vi "ConnRecoveryThread.vi"(0 "reference in":refnum<class "SuperNS.lvclass">) -> ()   [LabVIEW 2020, in "SuperNS.lvclass"]
doc: "Copyright © 2008 - 2024 VI Technologies B.V. \nALL RIGHTS RESERVED"
uses:
  SuperNS.lvclass
  StreamDataType.ctl
  <vilib>/dex/Flush And Wait Empty Condition.ctl
  <vilib>/Utility/error.llb/Error Cluster From Error Code.vi
  <vilib>/ErrorRing/Error Ring.xnode
  SuperNS.lvclass/SuperNS.ctl
  <resource>/objmgr/ni.dex.rc
panel:
  out "Disconnected timeout":bool
  out "Is Connected":bool
  out "Remote Endpoint Destroyed":bool
  out "Last error":errorcluster
  out "IsWriterEndpoint":bool
  out "Iteration":i32
  # "Copyright (c) 2024, VI Technologies B.V.\nAll rights reserved.\n\nRedistribution and use in source and binary forms, with or without modification, are permitted provided that \nthe following conditions are met:\n\n * Redistributions of source code must retain the above copyright notice, this list of conditions and the \nfollowing disclaimer.\n * Redistributions in binary form must reproduce the above copyright notice, this list of conditions and the \nfollowing disclaimer in the documentation and/or other materials provided with the distribution.\n * Neither the name of VI Technologies B.V. nor the names of its contributors may be used to endorse or \npromote products derived from this software without specific prior written permission.\n\nTHIS SOFTWARE IS PROVIDED BY THE COPYRIGHT HOLDERS AND CONTRIBUTORS \"AS IS\" AND ANY EXPRESS OR \nIMPLIED WARRANTIES, INCLUDING, BUT NOT LIMITED TO, THE IMPLIED WARRANTIES OF MERCHANTABILITY \nAND FITNESS FOR A PARTICULAR PURPOSE ARE DISCLAIMED. IN NO EVENT SHALL THE COPYRIGHT OWNER OR \nCONTRIBUTORS BE LIABLE FOR ANY DIRECT, INDIRECT, INCIDENTAL, SPECIAL, EXEMPLARY, OR CONSEQUENTIAL \nDAMAGES (INCLUDING, BUT NOT LIMITED TO, PROCUREMENT OF SUBSTITUTE GOODS OR SERVICES; LOSS OF \nUSE, DATA, OR PROFITS; OR BUSINESS INTERRUPTION) HOWEVER CAUSED AND ON ANY THEORY OF LIABILITY, \nWHETHER IN CONTRACT, STRICT LIABILITY, OR TORT (INCLUDING NEGLIGENCE OR OTHERWISE) ARISING IN ANY \nWAY OUT OF THE USE OF THIS SOFTWARE, EVEN IF ADVISED OF THE POSSIBILITY OF SUCH DAMAGE.\n\nFor more information, please visit https://www.vi-tech.nl or contact us at info@vi-tech.nl"
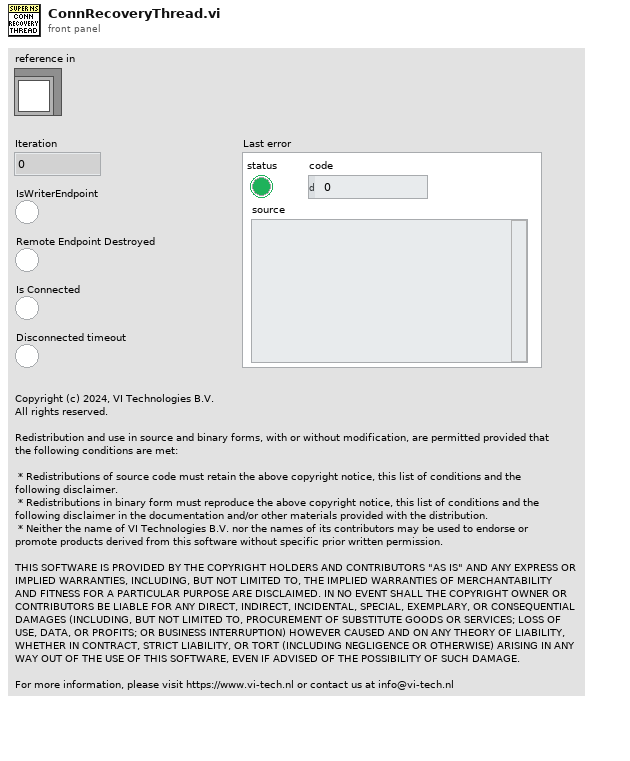
[diagram p1: front panel]
types:
  T1 = typedef "SuperNS.lvclass/ObjectAttributes.ctl" = cluster{"NSName":string, "RemoteEP_URL":string, "BufferSize":i32, "Element Allocation Mode":T2, "ConnLost Timeout":i32, "Writer":bool, "ReadDataEvent":string, "FlushAfterWrite":bool, "Thread":cluster{"VI Refnum":refnum<vi>, "Started Notifier":refnum<notifier>, "Stopped Notifier":refnum<notifier>, "CmdEvent":refnum<user-event>}, "Endpoint":refnum<k21>, "R/W Error":bool, "Flush Wait Condition":T3, "DataReadEvent":refnum<user-event>, "NS Created":bool, "BG ConnCheck/Read period":i32, "ErrorEvent":refnum<user-event>}
  T2 = typedef "Stream Element Allocation Mode.ctl" = u32
  T3 = typedef "Flush And Wait Empty Condition.ctl" = u8
  T4 = typedef "SuperNS.lvclass/StreamDataType.ctl" = refnum<class>
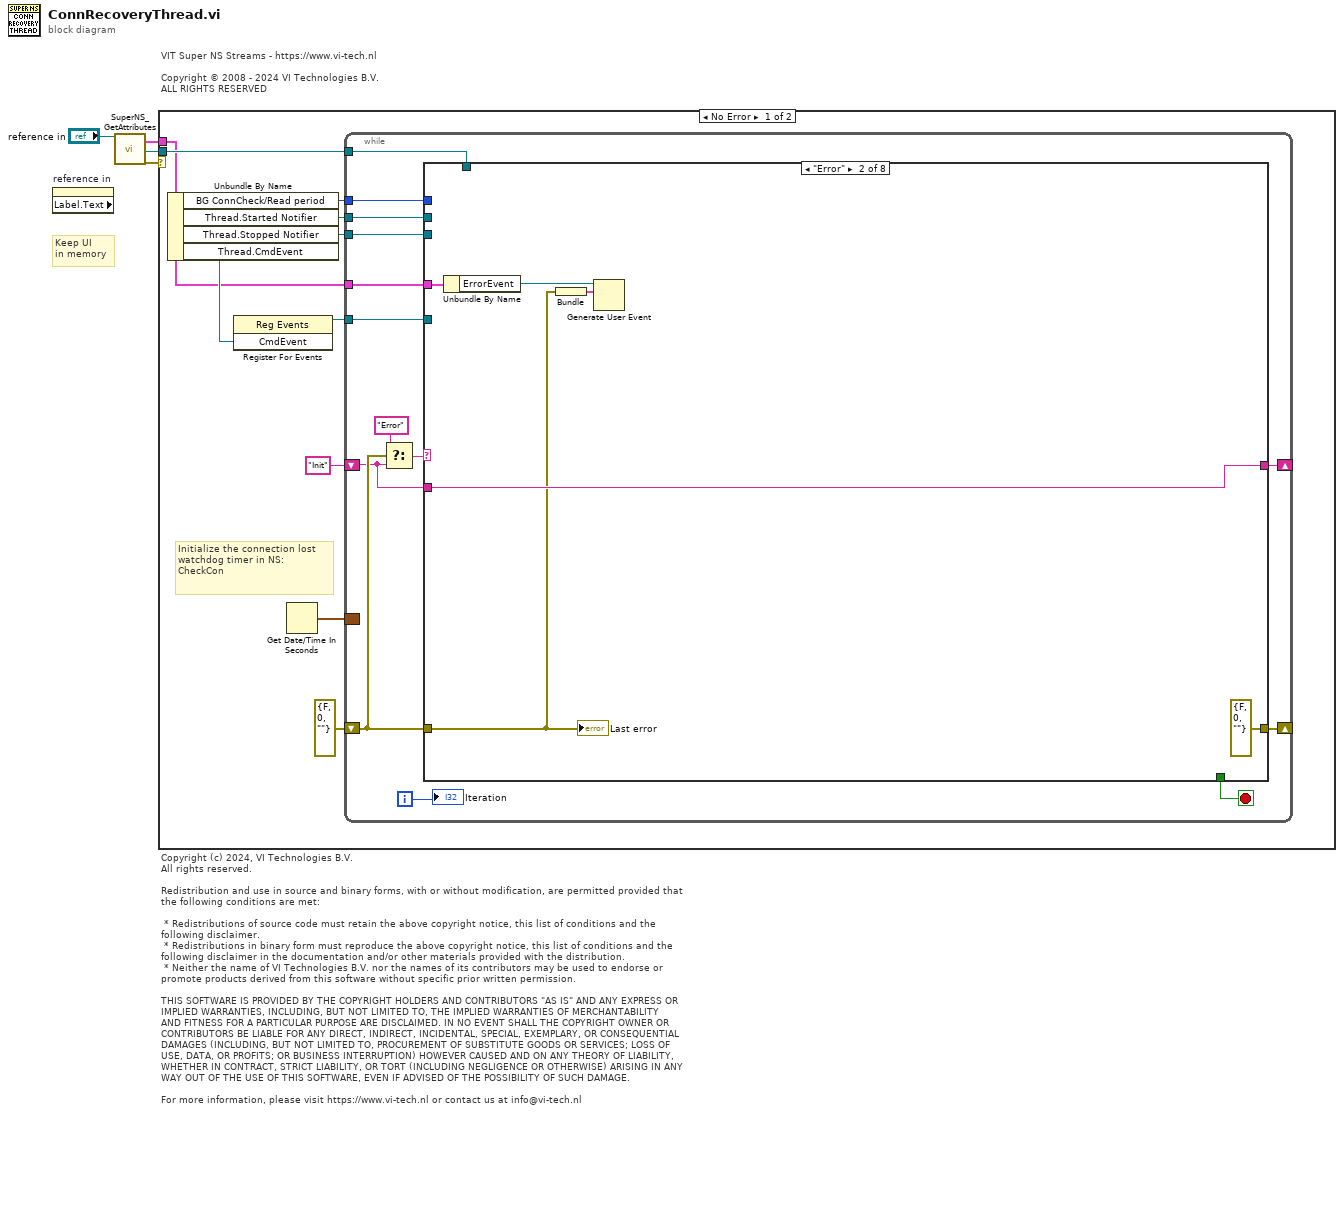
[diagram p0: block diagram]
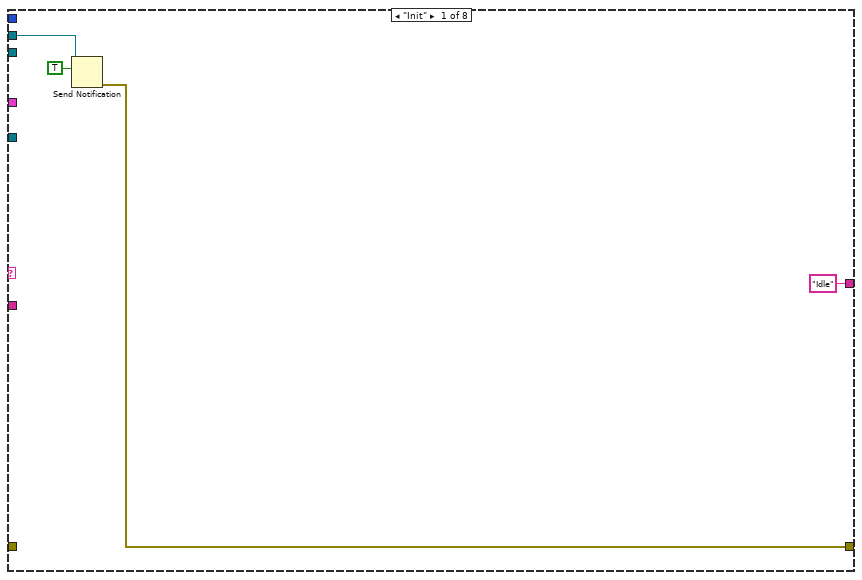
[diagram p2: hidden frame]
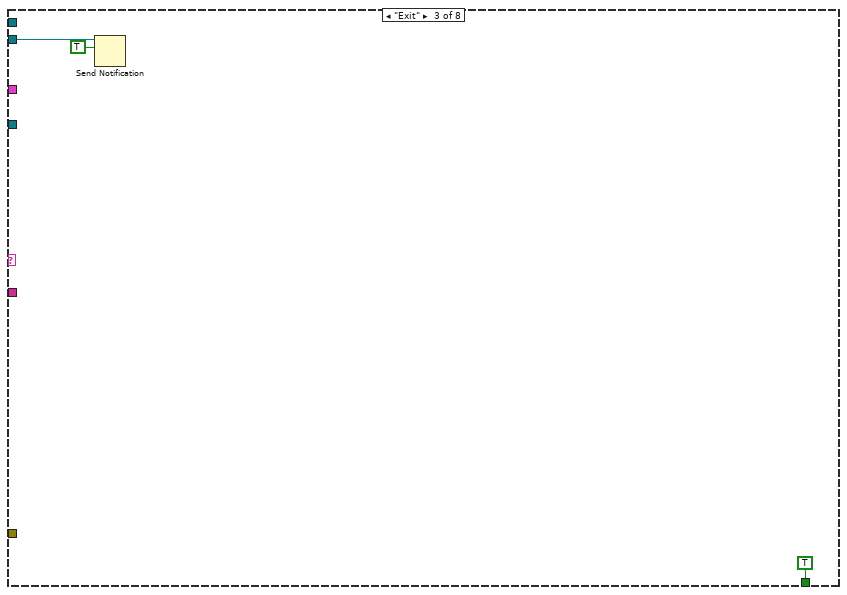
[diagram p3: hidden frame]
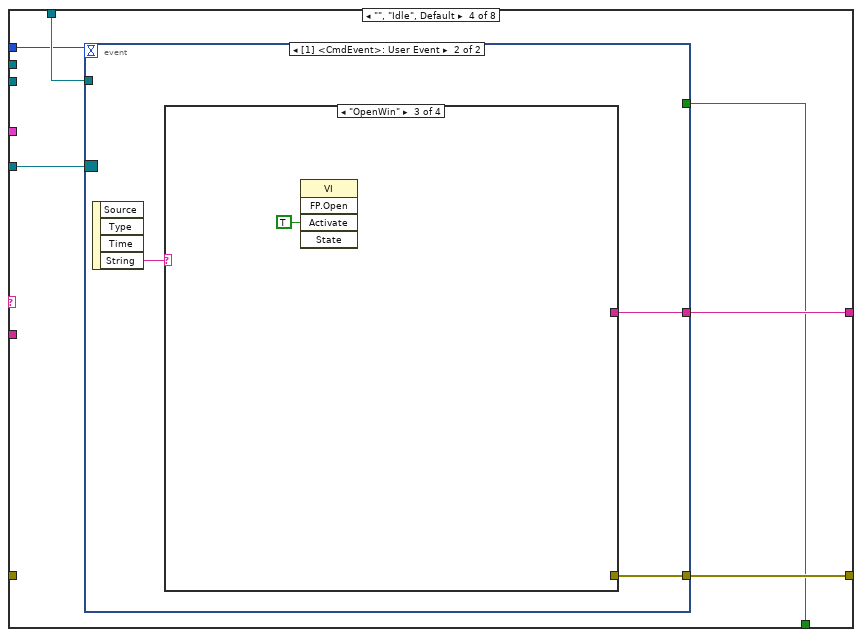
[diagram p4: hidden frame]
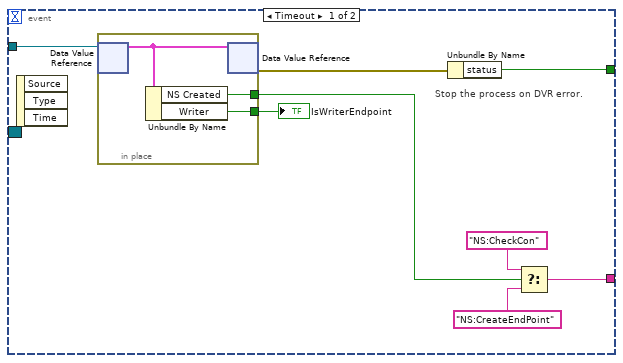
[diagram p5: hidden frame]
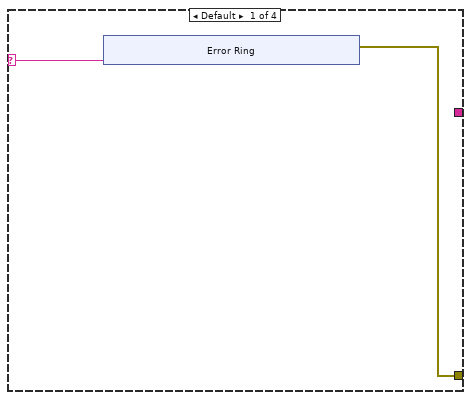
[diagram p6: hidden frame]
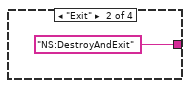
[diagram p7: hidden frame]
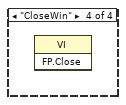
[diagram p8: hidden frame]
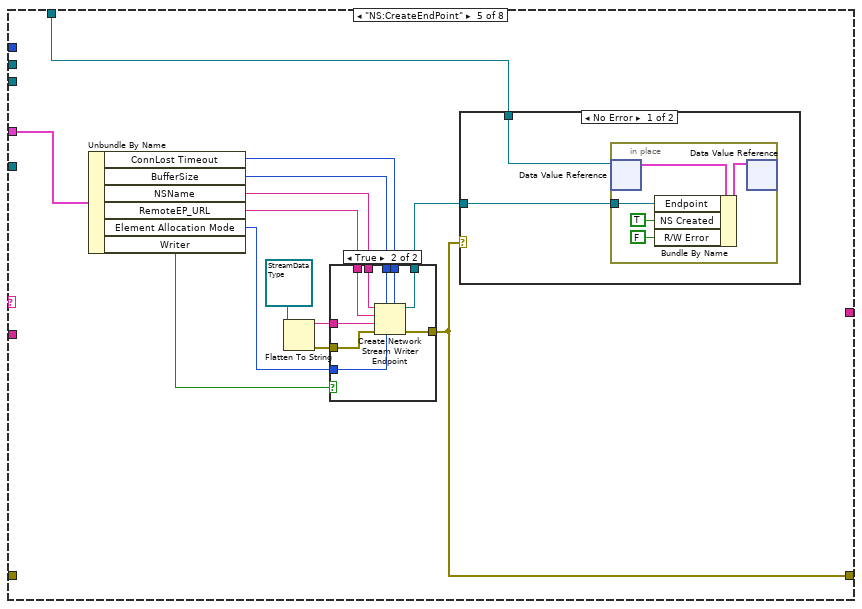
[diagram p9: hidden frame]
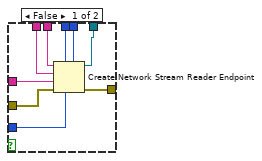
[diagram p10: hidden frame]
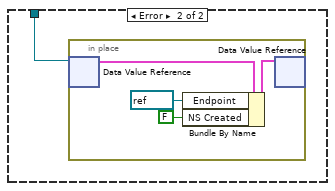
[diagram p11: hidden frame]
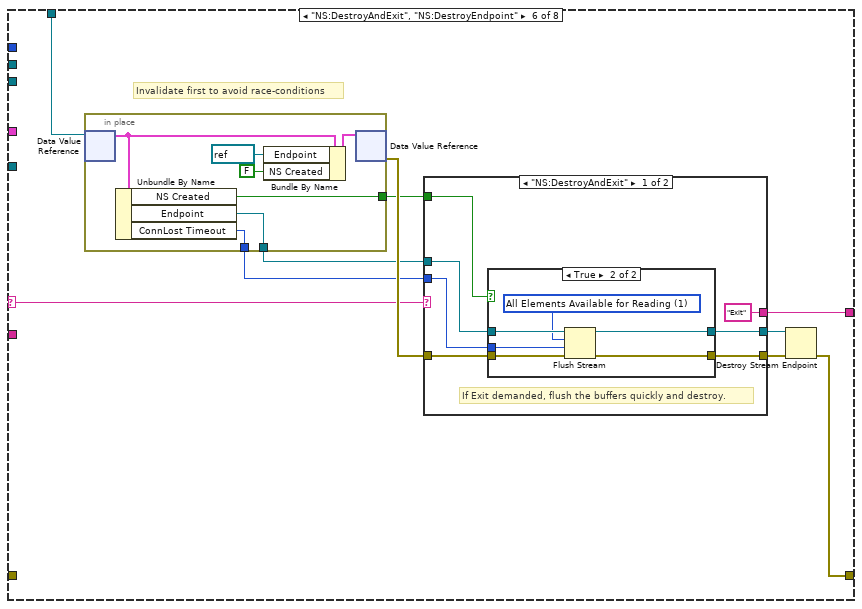
[diagram p12: hidden frame]
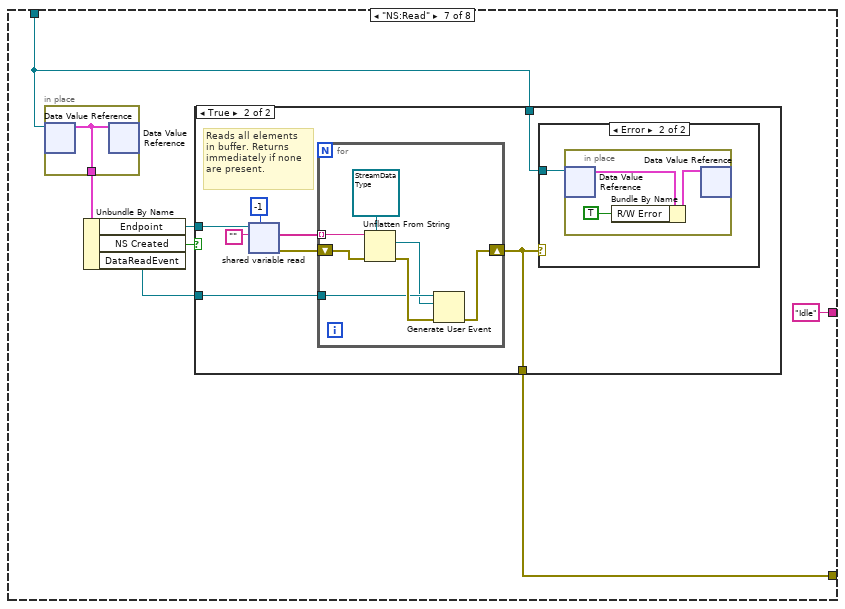
[diagram p15: hidden frame]
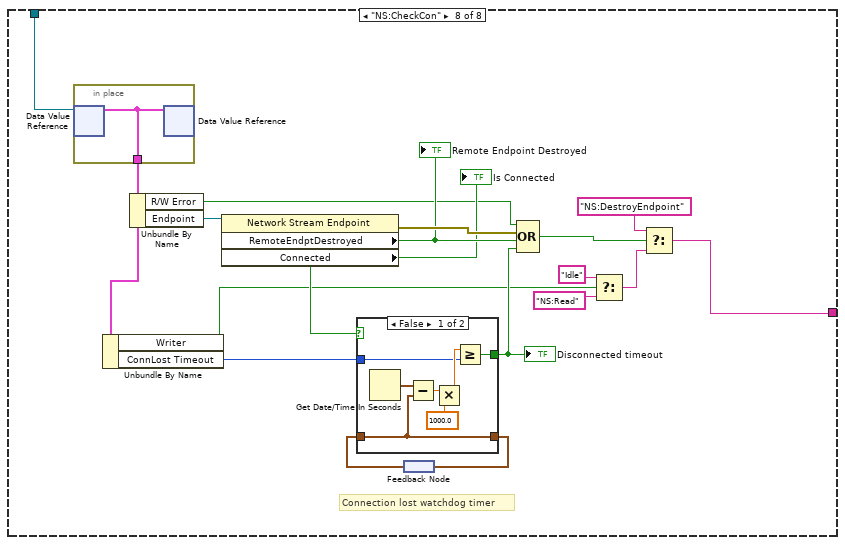
[diagram p18: hidden frame]
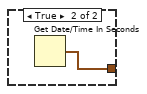
[diagram p19: hidden frame]
diagram:
  # "VIT Super NS Streams - https://www.vi-tech.nl\n\nCopyright © 2008 - 2024 VI Technologies B.V. \nALL RIGHTS RESERVED"
  # "Copyright (c) 2024, VI Technologies B.V.\nAll rights reserved.\n\nRedistribution and use in source and binary forms, with or without modification, are permitted provided that \nthe following conditions are met:\n\n * Redistributions of source code must retain the above copyright notice, this list of conditions and the \nfollowing disclaimer.\n * Redistributions in binary form must reproduce the above copyright notice, this list of conditions and the \nfollowing disclaimer in the documentation and/or other materials provided with the distribution.\n * Neither the name of VI Technologies B.V. nor the names of its contributors may be used to endorse or \npromote products derived from this software without specific prior written permission.\n\nTHIS SOFTWARE IS PROVIDED BY THE COPYRIGHT HOLDERS AND CONTRIBUTORS \"AS IS\" AND ANY EXPRESS OR \nIMPLIED WARRANTIES, INCLUDING, BUT NOT LIMITED TO, THE IMPLIED WARRANTIES OF MERCHANTABILITY \nAND FITNESS FOR A PARTICULAR PURPOSE ARE DISCLAIMED. IN NO EVENT SHALL THE COPYRIGHT OWNER OR \nCONTRIBUTORS BE LIABLE FOR ANY DIRECT, INDIRECT, INCIDENTAL, SPECIAL, EXEMPLARY, OR CONSEQUENTIAL \nDAMAGES (INCLUDING, BUT NOT LIMITED TO, PROCUREMENT OF SUBSTITUTE GOODS OR SERVICES; LOSS OF \nUSE, DATA, OR PROFITS; OR BUSINESS INTERRUPTION) HOWEVER CAUSED AND ON ANY THEORY OF LIABILITY, \nWHETHER IN CONTRACT, STRICT LIABILITY, OR TORT (INCLUDING NEGLIGENCE OR OTHERWISE) ARISING IN ANY \nWAY OUT OF THE USE OF THIS SOFTWARE, EVEN IF ADVISED OF THE POSSIBILITY OF SUCH DAMAGE.\n\nFor more information, please visit https://www.vi-tech.nl or contact us at info@vi-tech.nl"
  # "Keep UI\nin memory"
  n1 = property on="reference in" class="LVClassControl (strict)" props=["Label", "Text"]() -> ()  [unwired: 2 in, 3 out]
  n2 = call "SuperNS_GetAttributes.vi"("reference in"="reference in") -> ("Data"=w1:T1, "DataRef"=w2:refnum<data-value>, "error out"=w4:errorcluster)  [unwired: 15 in, 1 out]
  n3 = case shown="No Error" w4 {
    tunnel: w1 -> [w5 _]
    tunnel: w2 -> [w8 _]
    frame No Error {
      # "Initialize the connection lost watchdog timer in NS: CheckCon"
      n4 = Unbundle By Name(w5) -> ("BG ConnCheck/Read period"=w7:i32, "Thread.Started Notifier"=w9:refnum<notifier>, "Thread.Stopped Notifier"=w11:refnum<notifier>, "Thread.CmdEvent"=w13:refnum<user-event>)
      n5 = register-events(w13) -> (reference out=w12:refnum<event-registration>)  [unwired: 2 in, 1 out]
      n6 = Get Date/Time In Seconds() -> (seconds since 1Jan1904=w6:timestamp)
      n7 = while {
        tunnel: w12 -> [w26]
        tunnel: w11 -> [w25]
        shift-right: [w19] -> _
        shift-left: "Init" -> [w18]
        tunnel: w9 -> [w22]
        shift-right: [w28] -> _
        shift-left: errorcluster {"status"=FALSE, "code"=0, "source"=""} ("error IO") -> [w27]
        tunnel: w8 -> [w17]
        tunnel: w5 -> [w16]
        tunnel: w7 -> [w15]
        border: w6 -> [_]
        i -> [w23]
        stop <- w24 stop-if-true
        n8 = Select(t="Error", s=w27, f=w18) -> (s? t:f=w21:string)
        n9 = case shown="\"Error\"" w21 {
          selector: w21 -> [_ _ _ _ _ w121 _ _]
          tunnel: w26 -> [_ _ _ w46 _ _ _ _]
          tunnel: w25 -> [_ _ w39 _ _ _ _ _]
          tunnel: [_ _ TRUE w42 _ _ _ _] -> w24
          tunnel: w22 -> [w30 _ _ _ _ _ _ _]
          tunnel: [w32 errorcluster {"status"=FALSE, "code"=0, "source"=""} ("error out") _ w47 w84 w123 w156 _] -> w28
          tunnel: ["Idle" w37 _ w45 _ w120 "Idle" w179] -> w19
          tunnel: w18 -> [_ w37 _ _ _ _ _ _]
          tunnel: w17 -> [_ _ _ w44 w73 w119 w151 w178]
          tunnel: w16 -> [_ w36 _ _ w75 _ _ _]
          tunnel: w27 -> [_ w33 _ _ _ _ _ _]
          tunnel: w15 -> [_ _ _ w43 _ _ _ _]
          frame "Init" {
            n10 = Send Notification(notification=TRUE, notifier=w30) -> (error out=w32:errorcluster)  [unwired: 1 in, 1 out]
          }
          frame "Error" {
            n11 = Unbundle By Name(w36) -> ("ErrorEvent"=w35:refnum<user-event>)
            n12 = Bundle("error IO"=w33) -> (w34:cluster{"error IO":errorcluster})  [unwired: 1 in]
            n13 = Generate User Event(user event=w35, event data cluster=w34) -> ()  [unwired: 2 in, 2 out]
            "Last error" <- w33
          }
          frame "Exit" {
            n14 = Send Notification(notification=TRUE, notifier=w39) -> ()  [unwired: 1 in, 2 out]
          }
          frame "", "Idle", Default {
            n15 = event shown="[1] <CmdEvent>: User Event" {
              selector: w46 -> [_ _]
              dyn-events: _ -> [_ _]
              timeout: w43 -> [_ _]
              tunnel: [_ w61] -> w47
              tunnel: [w52 w59] -> w45
              tunnel: w44 -> [w51 _]
              tunnel: [w48 _] -> w42
              event Timeout {
                # "Stop the process on DVR error."
                n16 = event-data() -> ()  [unwired: 1 in, 3 out]
                n17 = in-place {
                  in-place-border: [w57] -> w50
                  in-place-border: [w56] -> w49
                  n18 = in-place-dvr #1(w51) -> (w58:T1)  [unwired: 1 out]
                  n19 = Unbundle By Name(w58) -> ("NS Created"=w57:bool, "Writer"=w56:bool)
                  n20 = in-place-dvr #1(w58) -> (w55:errorcluster)  [unwired: 1 out]
                }
                "IsWriterEndpoint" <- w49
                n21 = Unbundle By Name(w55) -> ("status"=w48:bool)
                n22 = Select(t="NS:CheckCon", s=w50, f="NS:CreateEndPoint") -> (s? t:f=w52:string)
              }
              event User Event {
                n23 = event-data() -> ("String"=w60:string)  [unwired: 1 in, 3 out]
                n24 = case shown="\"OpenWin\"" w60 {
                  selector: w60 -> [w62 _ _ _]
                  tunnel: [w63 _ _ _] -> w61
                  tunnel: [_ "NS:DestroyAndExit" _ _] -> w59
                  frame Default {
                    n25 = xnode "Error Ring"("parameter 0"=w62) -> ("error out"=w63:errorcluster)
                  }
                  frame "Exit" {
                  }
                  frame "OpenWin" {
                    n26 = invoke class="VI" method="FP.Open"("Activate"=TRUE ("Activate?")) -> ()  [unwired: 4 in, 5 out]
                  }
                  frame "CloseWin" {
                    n27 = invoke class="VI" method="FP.Close"() -> ()  [unwired: 3 in, 3 out]
                  }
                }
              }
            }
          }
          frame "NS:CreateEndPoint" {
            n28 = Unbundle By Name(w75) -> ("ConnLost Timeout"=w80:i32, "BufferSize"=w79:i32, "NSName"=w82:string, "RemoteEP_URL"=w81:string, "Element Allocation Mode"=w78:T2, "Writer"=w76:bool)
            n29 = Flatten To String(anything=T4 refnum ("LabVIEW Object")) -> (data string=w83:string, error out=w85:errorcluster)  [unwired: 3 in, 1 out]
            n30 = case shown="True" w76 {
              tunnel: w83 -> [w86 w101]
              tunnel: w85 -> [w93 w103]
              tunnel: w82 -> [w91 w100]
              tunnel: w81 -> [w90 w99]
              tunnel: w80 -> [w88 w98]
              tunnel: w79 -> [w89 w97]
              tunnel: w78 -> [w92 w96]
              tunnel: [w94 w102] -> w84
              tunnel: [w87 w95] -> w77
              frame False {
                n31 = Create Network Stream Reader Endpoint(5:w88, 6:w92, 7:w89, 8:w93, 9:w86, 10:w90, 11:w91) -> (0:w94:errorcluster, 3:w87:refnum<k21>)
              }
              frame True {
                n32 = Create Network Stream Writer Endpoint(5:w98, 6:w96, 7:w97, 8:w103, 9:w101, 10:w99, 11:w100) -> (0:w102:errorcluster, 3:w95:refnum<k21>)
              }
            }
            n33 = case shown="No Error" w84 {
              tunnel: w77 -> [w104 _]
              tunnel: w73 -> [w105 w111]
              frame No Error {
                n34 = in-place {
                  in-place-border: w104 -> [w106]
                  n35 = in-place-dvr #2(w105) -> (w110:T1)  [unwired: 1 out]
                  n36 = Bundle By Name(cluster=w110, "Endpoint"=w106, "NS Created"=TRUE, "R/W Error"=FALSE) -> (w109:T1)
                  n37 = in-place-dvr #2(w109) -> ()  [unwired: 2 out]
                }
              }
              frame Error {
                n38 = in-place {
                  n39 = in-place-dvr #3(w111) -> (w115:T1)  [unwired: 1 out]
                  n40 = Bundle By Name(cluster=w115, "Endpoint"=refnum<k21> refnum, "NS Created"=FALSE) -> (w114:T1)
                  n41 = in-place-dvr #3(w114) -> ()  [unwired: 2 out]
                }
              }
            }
          }
          frame "NS:DestroyAndExit", "NS:DestroyEndpoint" {
            # "Invalidate first to avoid race-conditions"
            n42 = in-place {
              in-place-border: [w145] -> w118
              in-place-border: [w144] -> w117
              in-place-border: [w143] -> w116
              n43 = in-place-dvr #4(w119) -> (w146:T1)  [unwired: 1 out]
              n44 = Unbundle By Name(w146) -> ("NS Created"=w143:bool, "Endpoint"=w145:refnum<k21>, "ConnLost Timeout"=w144:i32)
              n45 = Bundle By Name(cluster=w146, "Endpoint"=refnum<k21> refnum, "NS Created"=FALSE) -> (w149:T1)
              n46 = in-place-dvr #4(w149) -> (w124:errorcluster)  [unwired: 1 out]
            }
            n47 = case shown="\"NS:DestroyAndExit\"" w121 {
              tunnel: w118 -> [w130 w141]
              tunnel: [w129 w141] -> w122
              tunnel: w117 -> [w128 _]
              tunnel: [w132 w142] -> w125
              tunnel: ["Exit" _] -> w120
              tunnel: w124 -> [w131 w142]
              tunnel: w116 -> [w126 _]
              frame "NS:DestroyAndExit" {
                # "If Exit demanded, flush the buffers quickly and destroy."
                n48 = case shown="True" w126 {
                  tunnel: w130 -> [w133 w138]
                  tunnel: [w133 w137] -> w129
                  tunnel: w128 -> [_ w135]
                  tunnel: [w134 w140] -> w132
                  tunnel: w131 -> [w134 w139]
                  frame False {
                    # "No need for flushing if there is\nno NS created."
                  }
                  frame True {
                    w136 = T3 1 items=["All Elements Read From Stream", "All Elements Available for Reading"] ("wait condition")
                    n49 = Flush Stream(8:w139, 9:w135, 10:w136, 11:w138) -> (0:w140:errorcluster, 3:w137:refnum<k21>)  [unwired: 1 out]
                  }
                }
              }
              frame "", Default {
              }
            }
            n50 = Destroy Stream Endpoint(8:w125, 11:w122) -> (0:w123:errorcluster)
          }
          frame "NS:Read" {
            n51 = in-place {
              in-place-border: [w157] -> w150
              n52 = in-place-dvr #5(w151) -> (w157:T1)  [unwired: 1 out]
              n53 = in-place-dvr #5(w157) -> ()  [unwired: 2 out]
            }
            n54 = Unbundle By Name(w150) -> ("Endpoint"=w155:refnum<k21>, "NS Created"=w153:bool, "DataReadEvent"=w154:refnum<user-event>)
            n55 = case shown="True" w153 {
              tunnel: w155 -> [_ w163]
              tunnel: w154 -> [_ w160]
              tunnel: w151 -> [_ w159]
              tunnel: [_ w164] -> w156
              frame False {
              }
              frame True {
                # "Reads all elements\nin buffer. Returns\nimmediately if none\nare present."
                n56 = shared-variable-read(w163, "", -1 ("# elements")) -> (w165:errorcluster, w161:string[])  [unwired: 2 in, 2 out]
                n57 = for {
                  tunnel: w161 -> [w173] mode=indexing
                  tunnel: w160 -> [w172]
                  shift-right: [w174] -> w164
                  shift-left: w165 -> [w176]
                  n58 = Unflatten From String(type=T4 refnum ("LabVIEW Object"), binary string=w173, error in (no error)=w176) -> (value=w171:T4, error out=w175:errorcluster)  [unwired: 2 in, 1 out]
                  n59 = Generate User Event(user event=w172, event data cluster=w171, error in=w175) -> (error out=w174:errorcluster)  [unwired: 1 in, 1 out]
                }
                n60 = case shown="Error" w164 {
                  tunnel: w159 -> [_ w166]
                  frame No Error {
                  }
                  frame Error {
                    n61 = in-place {
                      n62 = in-place-dvr #6(w166) -> (w169:T1)  [unwired: 1 out]
                      n63 = Bundle By Name(cluster=w169, "R/W Error"=TRUE) -> (w168:T1)
                      n64 = in-place-dvr #6(w168) -> ()  [unwired: 2 out]
                    }
                  }
                }
              }
            }
          }
          frame "NS:CheckCon" {
            # "Connection lost watchdog timer"
            n65 = in-place {
              in-place-border: [w195] -> w177
              n66 = in-place-dvr #7(w178) -> (w195:T1)  [unwired: 1 out]
              n67 = in-place-dvr #7(w195) -> ()  [unwired: 2 out]
            }
            n68 = Unbundle By Name(w177) -> ("Writer"=w184:bool, "ConnLost Timeout"=w188:i32)
            n69 = Unbundle By Name(w177) -> ("R/W Error"=w180:bool, "Endpoint"=w193:refnum<k21>)
            n70 = property class="Network Stream Endpoint"(reference=w193) -> (error out=w194:errorcluster, "RemoteEndptDestroyed"=w192:bool, "Connected"=w191:bool)  [unwired: 1 in, 1 out]
            "Remote Endpoint Destroyed" <- w192
            "Is Connected" <- w191
            n71 = feedback #8() -> (w189:timestamp)
            n72 = case shown="False" w191 {
              tunnel: [w199 w203] -> w190
              tunnel: w189 -> [w199 _]
              tunnel: w188 -> [w197 _]
              tunnel: [w196 _] -> w187
              frame False {
                n73 = Get Date/Time In Seconds() -> (seconds since 1Jan1904=w202:timestamp)
                n74 = Subtract(x=w202, y=w199) -> (x-y=w201:dbl)
                n75 = Multiply(x=w201, y=1000.0) -> (x*y=w198:dbl)
                n76 = Greater Or Equal?(x=w198, y=w197) -> (x >= y?=w196:bool)
              }
              frame True {
                n77 = Get Date/Time In Seconds() -> (seconds since 1Jan1904=w203:timestamp)
              }
            }
            "Disconnected timeout" <- w187
            n78 = feedback-in #8(w190) -> ()
            n79 = Compound Arithmetic op=OR ("OR")(w180, w194, w192, w187) -> (w185:bool)
            n80 = Select(t="Idle", s=w184, f="NS:Read") -> (s? t:f=w182:string)
            n81 = Select(t="NS:DestroyEndpoint", s=w185, f=w182) -> (s? t:f=w179:string)
          }
        }
        "Iteration" <- w23
      }
    }
    frame Error {
    }
  }
